vi "modbusRTU.vi"() -> ()   [LabVIEW 2019]
uses:
  <vilib>/Modbus/master/Create Master Instance (Serial).vi
  <vilib>/Modbus/master/Modbus Master.lvclass
panel:
  in  "Limpar":bool
  out "?":T1(graph)
  in  "Reset Button":bool
  out "modo (short)":enum16{"short", "long"}(ring) caption="Modo (16 ou 32b)"
  out "sistema 01":enum16{"sistema 01"}(ring) caption="Tipo do sistema"
  out "freq nom":enum16{"50 hz", "60 hz"}(ring) caption="Freq nominal"
  out "formato dado":T2(ring) caption="Formato dado"
  out "polaridade tc":enum16{"(+)", "(-)"}(ring) caption="Polaridade sensor"
  out "Gauge 2 Baud rate":u16(knob) caption="Baud rate" scale=1.0..8.0
  out "Freq instântanea":sgl
  out "Energia ativa total":sgl caption="Energia total kWh" format="%#.4f"
  out "Pot aparente fase A":sgl
  out "Pot reativa fase A":sgl
  out "Pot ativa fase A":sgl
  out "FP fase A":sgl
  out "Corrente fase A":sgl
  out "Tensão fase A":sgl
  out "estado saida IO2":bool caption="Estado saída I/O2"
  in  "holding register value input":u16 caption="Valor\nholding register"
  in  "holding register address":u16(ring) caption="Endereço\nholding register" items=["SPLL"=26, "SPHL"=27, "Type"=43, "Ctrl"=46, "Act"=48, "Atun"=49, "Unit"=67]
  out "SPHL":dbl
  out "SPLL":dbl
  in  "Write Button":bool
  out "Horizontal Pointer Slide Pb":dbl caption="Pb"
  out "Horizontal Pointer Slide Ir":dbl caption="Ir"
  out "Horizontal Pointer Slide 1 Dt":dbl caption="Dt"
  in  "Boolean Run":bool caption="Run"
  out "Gauge Baud rate":u16(knob) caption="Baud rate" scale=0.0..6.0
  in  "exit button":bool
  out "unit ID (nó)":u16 caption="Unit ID (nó)"
  out "Thermometer PV":dbl(slide) caption="PV - Temperatura" scale=0.0..300.0
  out "Unit":enum16{"ºC", "ºF"}(ring)
  out "Atun":T3(ring)
  out "Act":enum16{"rE", "d Ir", ""}(ring)
  out "Run":u16
  out "Ctrl":enum16{"Man", "Auto"}(ring)
  out "Addr (nó)":u16
  out "Type sensor":enum16{"", "tc K"}(ring) caption="Type"
  out "MV":u16(slide) caption="MV \n   ação \n     de \ncontrole" scale=0.0..100.0
  in  "stop button":bool
  in  "start button":bool
  in  "modo Modbus":enum16{"RTU", "ASCII"}(ring)
  in  "VISA resource name \nCOM port":refnum<visa-resource-name>="COM4"
  in  "parity bit":u16(ring)=2 caption="bit de paridade" items=["None", "Odd", "Even"]
  in  "flow control":u16(ring) items=["None", "XON/XOFF", "RTS/CTS", "XON/XOFF & RTS/CTS", "DTR/DSR", "XON/XOFF & DTR/DSR"]
  in  "baud rate":u32(ring)=9600 items=["1200"=1200, "2400"=2400, "4800"=4800, "9600"=9600, "19200"=19200, "57600"=57600]
  in  "holding register value SP":u16 caption="Setpoint (SP)"
  # "COMUNICAÇÃO ON/OFF"
  # "CONTROLADOR PID N1200"
  # "MULTIMEDIDOR M-200"
  # "VALORES REFERÊNCIA"
  # "Reading holding \n    registers (03)"
  # "Reading input \n  registers (04)"
  # "167 ºC"
  # "220 Vca"
  # "0,13 A"
  # "FP 0,99"
  # "Writing single \n  registers (06)"
  # "*Valores de referência do sistema sem controle de temperatura"
  # "Reading coils (01)"
  # "MESTRE \nMODBUS  RTU"
  # "Reading holding registers (03)"
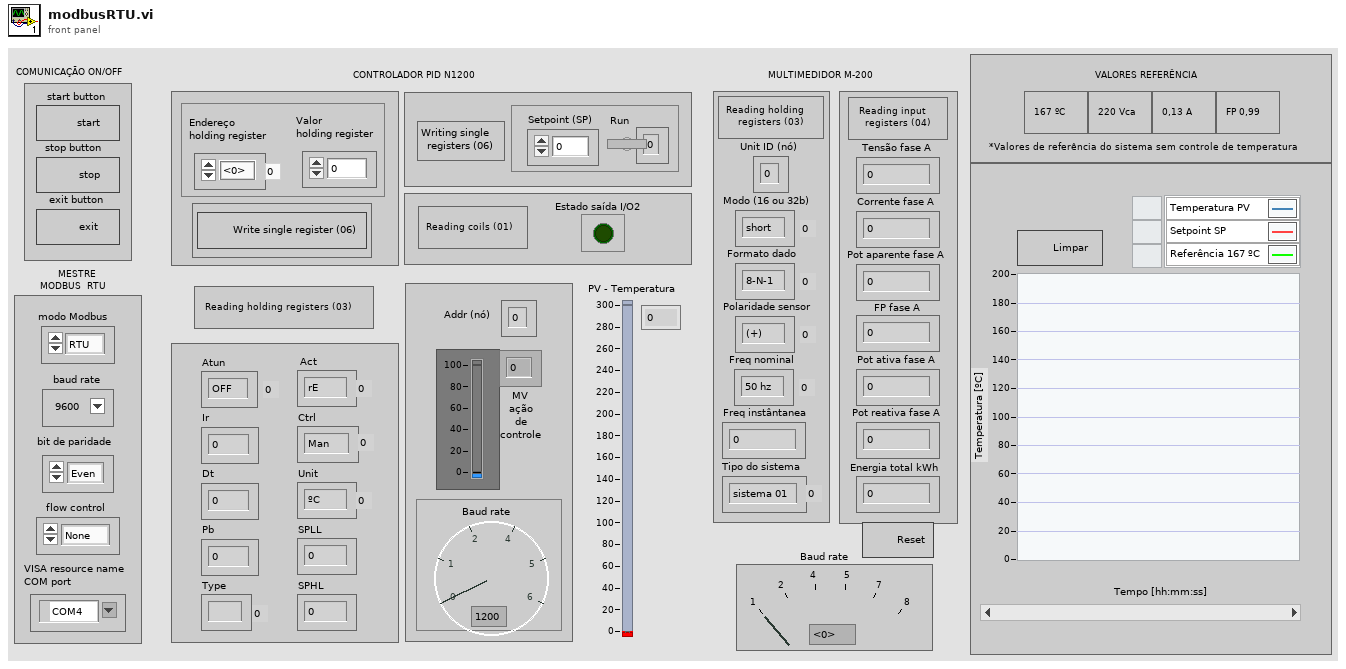
[diagram p1: front panel]
types:
  T1 = cluster{dbl, "y":u16, "holding register value SP":u16}
  T2 = enum16{"8-N-1", "8-N-2", "8-E-1", "8-E-2", "8-O-1", "8-O-2"}
  T3 = enum16{"OFF", "FAST", "FULL", "SELF", "RSELF", "TGHT"}
  T4 = cluster{dbl, "y":u16, "holding register value SP":u16}[]
  T5 = cluster{dbl, "holding register value SP":u16, "y":u16}
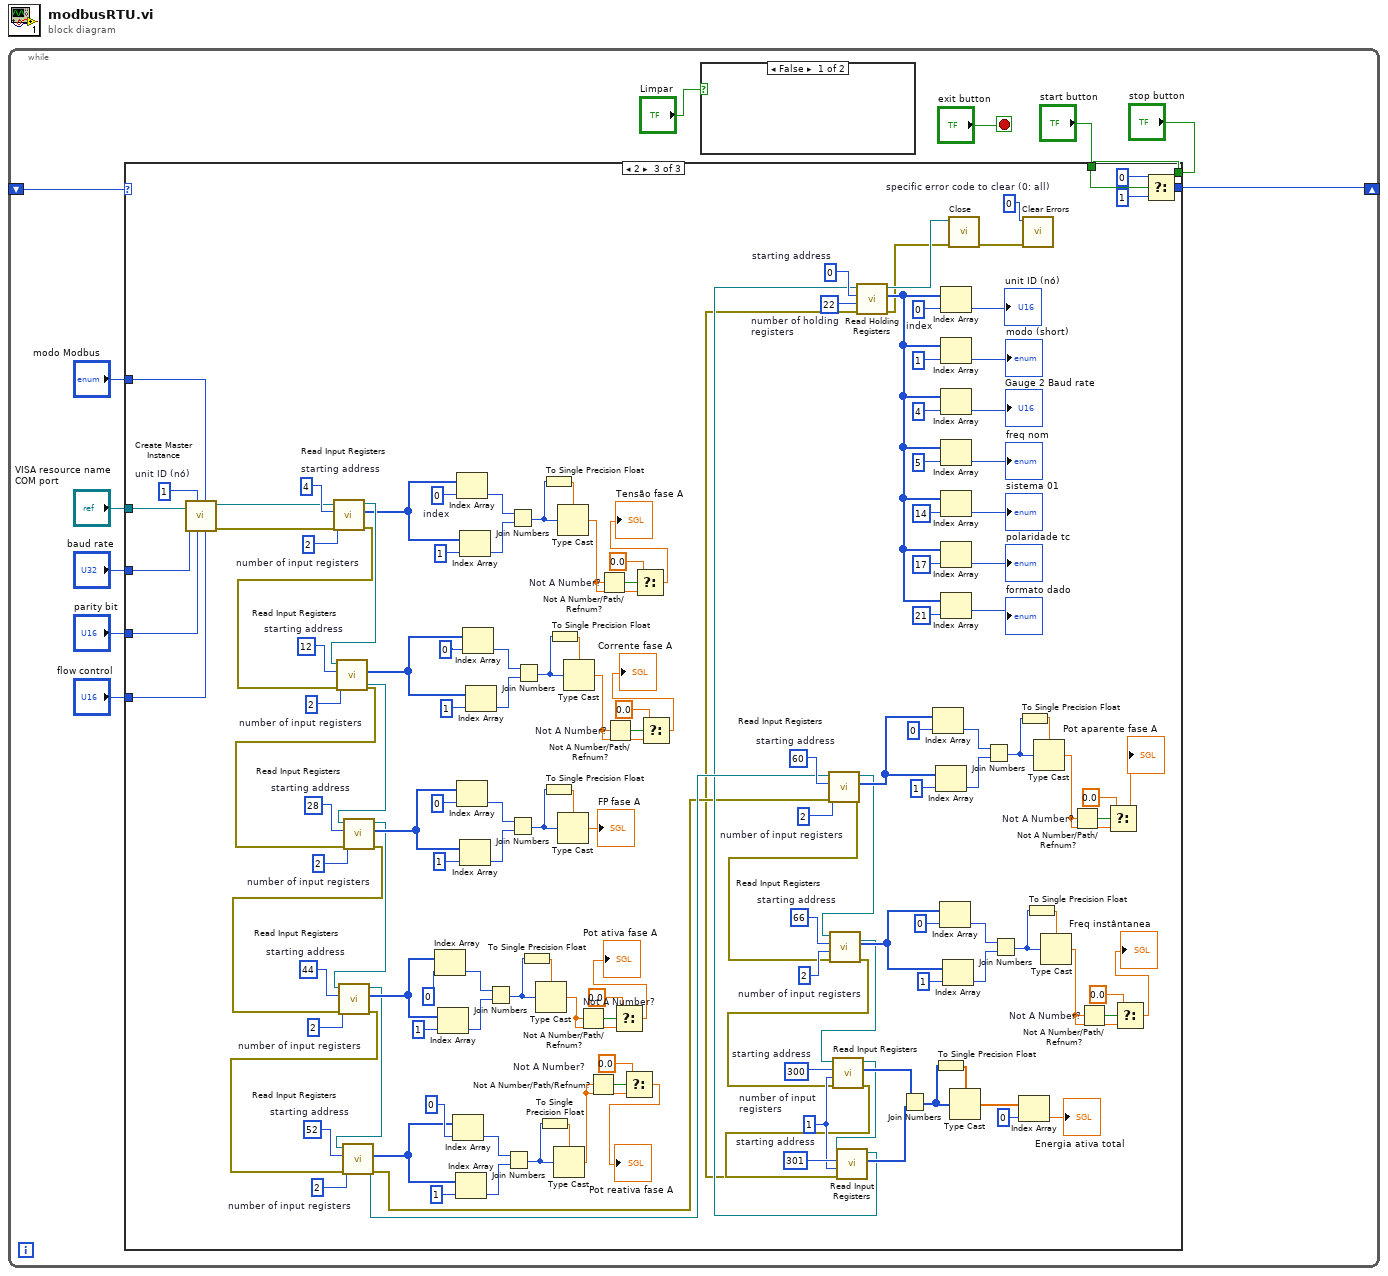
[diagram p0: block diagram]
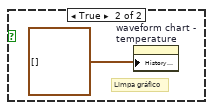
[diagram p2: hidden frame]
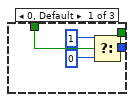
[diagram p3: hidden frame]
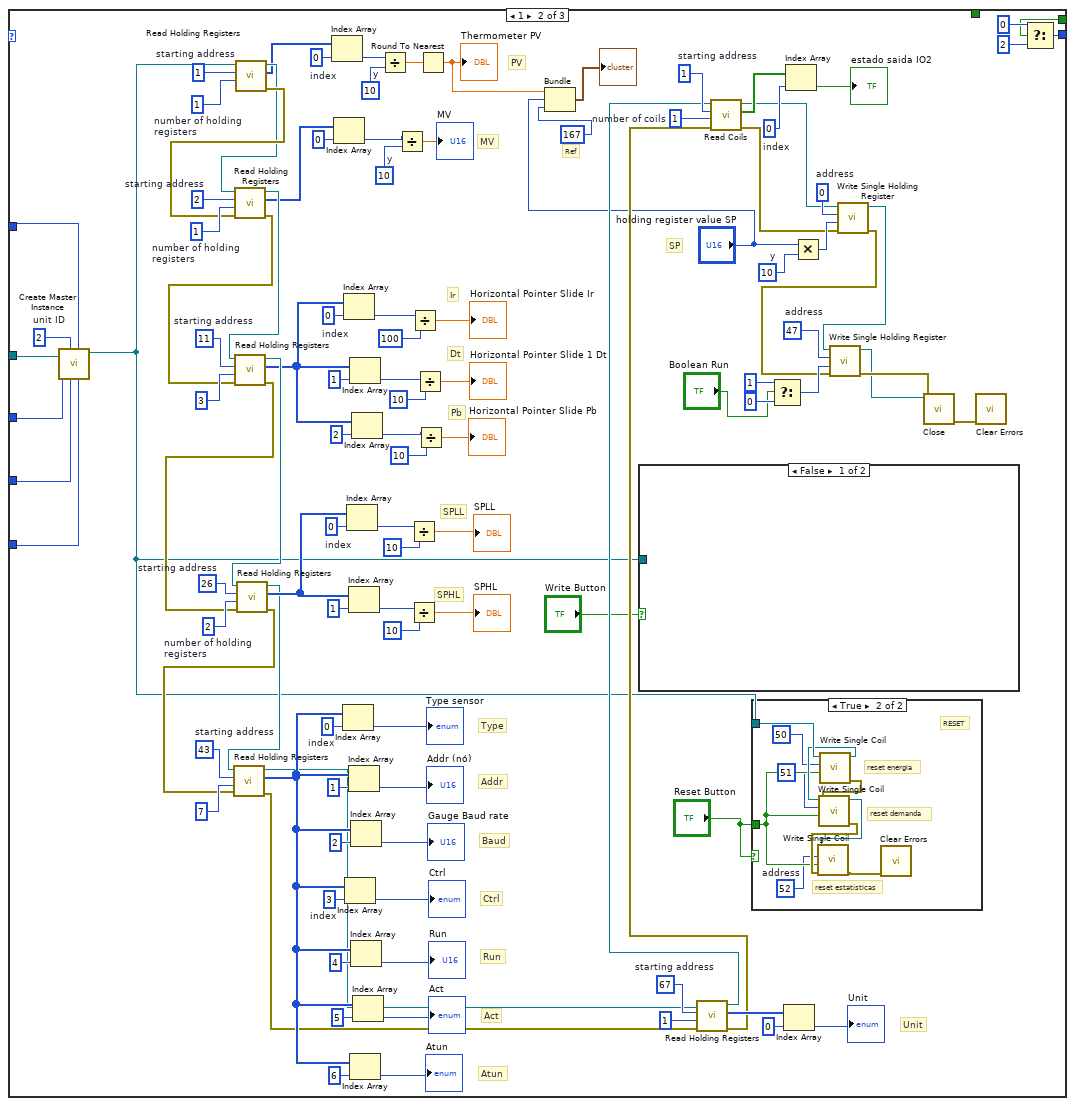
[diagram p4: hidden frame]
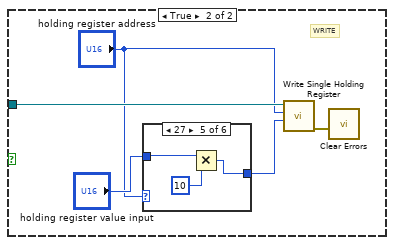
[diagram p6: hidden frame]
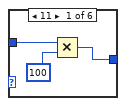
[diagram p7: hidden frame]
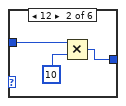
[diagram p8: hidden frame]
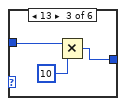
[diagram p9: hidden frame]
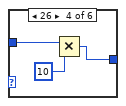
[diagram p10: hidden frame]
diagram:
  n1 = while {
    shift-right: [w10] -> _
    shift-left: _ -> [w11]
    stop <- "exit button" stop-if-true
    n2 = case shown="2" w11 {
      tunnel: [w16 w120 w303] -> w10
      tunnel: "stop button" -> [_ w119 w302]
      tunnel: "modo Modbus" -> [_ w118 w301]
      tunnel: "VISA resource name \nCOM port" -> [_ w117 w300]
      tunnel: "parity bit" -> [_ w115 w299]
      tunnel: "flow control" -> [_ w114 w298]
      tunnel: "baud rate" -> [_ w116 w297]
      tunnel: "start button" -> [w13 _ _]
      frame 0, Default {
        n3 = Select(t=1, s=w13, f=0) -> (s? t:f=w16:i32)
      }
      frame 1 {
        w29 = u16 1  # number of holding registers
        w30 = u16 1  # starting address
        w49 = 0  # index
        w52 = u16 1  # number of coils
        w53 = u16 1  # starting address
        w62 = u16 47  # address
        w66 = u16 10  # y
        w77 = u8 2  # unit ID
        w81 = u16 67  # starting address
        w91 = 3  # index
        w96 = 0  # index
        w98 = u16 43  # starting address
        w102 = 0  # index
        w99 = u16 2  # number of holding registers
        w103 = u16 26  # starting address
        w106 = 0  # index
        w108 = u16 11  # starting address
        w111 = 0  # index
        w112 = u16 10  # y
        w113 = u16 10  # y
        w125 = u16 1  # number of holding registers
        w126 = u16 2  # starting address
        w127 = u16 0  # address
        # "Ref"
        # "Unit"
        # "Atun"
        # "Act"
        # "Run"
        # "Ctrl"
        # "Baud"
        # "Addr"
        # "Type"
        # "SPHL"
        # "SPLL"
        # "Pb"
        # "Dt"
        # "Ir"
        # "MV"
        # "PV"
        # "SP"
        n4 = call-poly <vilib>:"Create Master Instance.vi"("flow control (None)"=w114, "serial type"=w118, "parity (Even)"=w115, "unit ID"=w77, "baud rate (9600)"=w116, "VISA resource name"=w117) -> ("serial master instance"=w22:refnum<class "Modbus Master.lvclass">)  [unwired: 4 in, 1 out]
        n5 = call-dynamic "Read Holding Registers.vi"("number of holding registers"=w29, "starting address"=w30, "Modbus master in"=w22) -> ("error out"=w28:errorcluster, "register values"=w23:u16[], "Modbus master out"=w27:refnum<class "Modbus Master.lvclass">)  [unwired: 6 in]
        n6 = call-dynamic "Read Holding Registers.vi"("error in (no error)"=w28, "number of holding registers"=w125, "starting address"=w126, "Modbus master in"=w27) -> ("error out"=w40:errorcluster, "register values"=w24:u16[], "Modbus master out"=w26:refnum<class "Modbus Master.lvclass">)  [unwired: 5 in]
        n7 = call-dynamic "Read Holding Registers.vi"("error in (no error)"=w40, "number of holding registers"=u16 3, "starting address"=w108, "Modbus master in"=w26) -> ("error out"=w39:errorcluster, "register values"=w25:u16[], "Modbus master out"=w46:refnum<class "Modbus Master.lvclass">)  [unwired: 5 in]
        n8 = call-dynamic "Read Holding Registers.vi"("error in (no error)"=w39, "number of holding registers"=w99, "starting address"=w103, "Modbus master in"=w46) -> ("error out"=w38:errorcluster, "register values"=w100:u16[], "Modbus master out"=w45:refnum<class "Modbus Master.lvclass">)  [unwired: 5 in]
        n9 = call-dynamic "Read Holding Registers.vi"("error in (no error)"=w38, "number of holding registers"=u16 7, "starting address"=w98, "Modbus master in"=w45) -> ("error out"=w37:errorcluster, "register values"=w83:u16[], "Modbus master out"=w44:refnum<class "Modbus Master.lvclass">)  [unwired: 5 in]
        n10 = Index Array "Index Array"(array=w23, index=w111) -> (element=w110:u16)
        n11 = Index Array(array=w24, index=0) -> (element=w65:u16)
        n12 = Index Array "Index Array"(array=w83, index=w96) -> (element=→"Type sensor":u16)
        n13 = Index Array "Index Array"(array=w25, index=w106) -> (element=w76:u16)
        n14 = Index Array(array=w83, index=w91) -> (element=→"Ctrl":u16)
        n15 = Index Array "Index Array"(array=w100, index=w102) -> (element=w69:u16)
        n16 = Index Array(array=w100, index=1) -> (element=w67:u16)
        n17 = Index Array(array=w83, index=1) -> (element=→"Addr (nó)":u16)
        n18 = Index Array(array=w25, index=1) -> (element=w73:u16)
        n19 = Index Array(array=w83, index=6) -> (element=→"Atun":u16)
        n20 = Index Array(array=w83, index=2) -> (element=→"Gauge Baud rate":u16)
        n21 = Index Array(array=w83, index=4) -> (element=→"Run":u16)
        n22 = Index Array(array=w25, index=2) -> (element=w71:u16)
        n23 = Index Array(array=w83, index=5) -> (element=→"Act":u16)
        n24 = Divide(x=w110, y=w112) -> (x/y=w123:dbl)
        n25 = Divide(x=w65, y=w66) -> (x/y=→"MV":dbl)
        n26 = Divide(x=w69, y=u16 10) -> (x/y=→"SPLL":dbl)
        n27 = Divide(x=w67, y=u16 10) -> (x/y=→"SPHL":dbl)
        n28 = Divide(x=w76, y=u16 100) -> (x/y=→"Horizontal Pointer Slide Ir":dbl)
        n29 = Divide(x=w73, y=u16 10) -> (x/y=→"Horizontal Pointer Slide 1 Dt":dbl)
        n30 = Divide(x=w71, y=u16 10) -> (x/y=→"Horizontal Pointer Slide Pb":dbl)
        n31 = Round To Nearest(number=w123) -> (nearest integer value=w20:dbl)
        "Thermometer PV" <- w20
        n32 = Bundle(w20, "holding register value SP"="holding register value SP", "y"=u16 167) -> (→"?":T5)  [unwired: 1 in]
        n33 = case shown="False" "Write Button" {
          tunnel: w22 -> [_ w141]
          frame False {
          }
          frame True {
            # "WRITE"
            n34 = case shown="27" "holding register address" {
              tunnel: [w144 w146 w149 w152 w155 w158] -> w140
              tunnel: "holding register value input" -> [w143 w147 w150 w153 w156 w158]
              frame 11 {
                n35 = Multiply(x=w143, y=u16 100) -> (x*y=w144:u16)
              }
              frame 12 {
                n36 = Multiply(x=w147, y=u16 10) -> (x*y=w146:u16)
              }
              frame 13 {
                n37 = Multiply(x=w150, y=u16 10) -> (x*y=w149:u16)
              }
              frame 26 {
                n38 = Multiply(x=w153, y=u16 10) -> (x*y=w152:u16)
              }
              frame 27 {
                n39 = Multiply(x=w156, y=u16 10) -> (x*y=w155:u16)
              }
              frame Default {
              }
            }
            n40 = call-dynamic "Write Single Holding Register.vi"("holding register value"=w140, "address"="holding register address", "Modbus master in"=w141) -> ("error out"=w142:errorcluster)  [unwired: 7 in, 1 out]
            n41 = call <vilib>:"Clear Errors.vi"("error in (no error)"=w142) -> ()  [unwired: 5 in, 2 out]
          }
        }
        n42 = call-dynamic "Read Holding Registers.vi"("error in (no error)"=w37, "number of holding registers"=u16 1, "starting address"=w81, "Modbus master in"=w44) -> ("error out"=w35:errorcluster, "register values"=w79:u16[], "Modbus master out"=w36:refnum<class "Modbus Master.lvclass">)  [unwired: 5 in]
        n43 = call-dynamic "Read Coils.vi"("error in (no error)"=w35, "number of coils"=w52, "starting address"=w53, "Modbus master in"=w36) -> ("error out"=w41:errorcluster, "coil values"=w50:bool[], "Modbus master out"=w47:refnum<class "Modbus Master.lvclass">)  [unwired: 5 in]
        n44 = case shown="True" "Reset Button" {
          tunnel: w22 -> [_ w134]
          tunnel: "Reset Button" -> [_ w131]
          frame False {
          }
          frame True {
            w130 = u16 52  # address
            # "RESET"
            # "reset estatísticas"
            # "reset demanda"
            # "reset energia"
            n45 = call-dynamic "Write Single Coil.vi"("coil value"=w131, "address"=u16 50, "Modbus master in"=w134) -> ("error out"=w137:errorcluster, "Modbus master out"=w133:refnum<class "Modbus Master.lvclass">)  [unwired: 7 in]
            n46 = call-dynamic "Write Single Coil.vi"("error in (no error)"=w137, "coil value"=w131, "address"=u16 51, "Modbus master in"=w133) -> ("error out"=w136:errorcluster, "Modbus master out"=w132:refnum<class "Modbus Master.lvclass">)  [unwired: 6 in]
            n47 = call-dynamic "Write Single Coil.vi"("error in (no error)"=w136, "coil value"=w131, "address"=w130, "Modbus master in"=w132) -> ("error out"=w135:errorcluster)  [unwired: 6 in, 1 out]
            n48 = call <vilib>:"Clear Errors.vi"("error in (no error)"=w135) -> ()  [unwired: 5 in, 2 out]
          }
        }
        n49 = Select(t=u16 1, s="Boolean Run", f=u16 0) -> (s? t:f=w59:u16)
        n50 = Index Array(array=w79, index=0) -> (element=→"Unit":u16)
        n51 = Index Array "Index Array"(array=w50, index=w49) -> (element=→"estado saida IO2":bool)
        n52 = Multiply(x="holding register value SP", y=w113) -> (x*y=w124:u16)
        n53 = call-dynamic "Write Single Holding Register.vi"("error in (no error)"=w41, "holding register value"=w124, "address"=w127, "Modbus master in"=w47) -> ("error out"=w42:errorcluster, "Modbus master out"=w51:refnum<class "Modbus Master.lvclass">)  [unwired: 6 in]
        n54 = call-dynamic "Write Single Holding Register.vi"("error in (no error)"=w42, "holding register value"=w59, "address"=w62, "Modbus master in"=w51) -> ("error out"=w34:errorcluster, "Modbus master out"=w33:refnum<class "Modbus Master.lvclass">)  [unwired: 6 in]
        n55 = call-dynamic "Close.vi"("error in (no error)"=w34, "Modbus master in"=w33) -> ("error out"=w43:errorcluster)  [unwired: 9 in]
        n56 = call <vilib>:"Clear Errors.vi"("error in (no error)"=w43) -> ()  [unwired: 5 in, 2 out]
        n57 = Select(t=0, s=w119, f=2) -> (s? t:f=w120:i32)
      }
      frame 2 {
        w189 = 0  # specific error code to clear (0: all)
        w222 = u16 2  # number of input registers
        w223 = u16 66  # starting address
        w228 = u16 2  # number of input registers
        w229 = u16 60  # starting address
        w230 = u16 2  # number of input registers
        w231 = u16 52  # starting address
        w232 = u16 2  # number of input registers
        w233 = u16 44  # starting address
        w234 = u16 2  # number of input registers
        w235 = u16 28  # starting address
        w236 = u16 2  # number of input registers
        w237 = u16 12  # starting address
        w246 = u16 301  # starting address
        w247 = u16 300  # starting address
        w238 = u16 1  # number of input registers
        w282 = 0  # index
        w285 = u16 2  # number of input registers
        w286 = u16 4  # starting address
        w294 = u8 1  # unit ID (nó)
        w296 = 0  # index
        w307 = u16 0  # starting address
        w306 = u16 22  # number of holding registers
        n58 = call-poly <vilib>:"Create Master Instance.vi"("flow control (None)"=w298, "serial type"=w301, "parity (Even)"=w299, "unit ID"=w294, "baud rate (9600)"=w297, "VISA resource name"=w300) -> ("error out"=w201:errorcluster, "serial master instance"=w203:refnum<class "Modbus Master.lvclass">)  [unwired: 4 in]
        n59 = call-dynamic "Read Input Registers.vi"("error in (no error)"=w201, "number of input registers"=w285, "starting address"=w286, "Modbus master in"=w203) -> ("error out"=w200:errorcluster, "register values"=w225:u16[], "Modbus master out"=w227:refnum<class "Modbus Master.lvclass">)  [unwired: 5 in]
        n60 = call-dynamic "Read Input Registers.vi"("error in (no error)"=w200, "number of input registers"=w236, "starting address"=w237, "Modbus master in"=w227) -> ("error out"=w199:errorcluster, "register values"=w212:u16[], "Modbus master out"=w226:refnum<class "Modbus Master.lvclass">)  [unwired: 5 in]
        n61 = call-dynamic "Read Input Registers.vi"("error in (no error)"=w199, "number of input registers"=w234, "starting address"=w235, "Modbus master in"=w226) -> ("error out"=w198:errorcluster, "register values"=w213:u16[], "Modbus master out"=w210:refnum<class "Modbus Master.lvclass">)  [unwired: 5 in]
        n62 = call-dynamic "Read Input Registers.vi"("error in (no error)"=w198, "number of input registers"=w232, "starting address"=w233, "Modbus master in"=w210) -> ("error out"=w197:errorcluster, "register values"=w214:u16[], "Modbus master out"=w209:refnum<class "Modbus Master.lvclass">)  [unwired: 5 in]
        n63 = call-dynamic "Read Input Registers.vi"("error in (no error)"=w197, "number of input registers"=w230, "starting address"=w231, "Modbus master in"=w209) -> ("error out"=w196:errorcluster, "register values"=w211:u16[], "Modbus master out"=w208:refnum<class "Modbus Master.lvclass">)  [unwired: 5 in]
        n64 = Index Array(array=w214, index=0) -> (element=w262:u16)
        n65 = Index Array(array=w214, index=1) -> (element=w260:u16)
        n66 = Index Array(array=w211, index=0) -> (element=w256:u16)
        n67 = Index Array(array=w211, index=1) -> (element=w254:u16)
        n68 = Index Array "Index Array"(array=w225, index=w282) -> (element=w281:u16)
        n69 = Index Array(array=w213, index=0) -> (element=w269:u16)
        n70 = Index Array(array=w225, index=1) -> (element=w279:u16)
        n71 = Index Array(array=w213, index=1) -> (element=w267:u16)
        n72 = Index Array(array=w212, index=0) -> (element=w275:u16)
        n73 = Index Array(array=w212, index=1) -> (element=w273:u16)
        n74 = Join Numbers(hi=w262, lo=w260) -> ((hi.lo)=w264:u32)
        n75 = Join Numbers(hi=w256, lo=w254) -> ((hi.lo)=w258:u32)
        n76 = Join Numbers(hi=w281, lo=w279) -> ((hi.lo)=w283:u32)
        n77 = Join Numbers(hi=w269, lo=w267) -> ((hi.lo)=w271:u32)
        n78 = Join Numbers(hi=w275, lo=w273) -> ((hi.lo)=w277:u32)
        n79 = To Single Precision Float(number=w264) -> (single precision float=w265:sgl)
        n80 = Type Cast(type=w265, x=w264) -> (*(type *) &x=w172:sgl)
        n81 = To Single Precision Float(number=w258) -> (single precision float=w259:sgl)
        n82 = To Single Precision Float(number=w283) -> (single precision float=w284:sgl)
        n83 = To Single Precision Float(number=w271) -> (single precision float=w272:sgl)
        n84 = To Single Precision Float(number=w277) -> (single precision float=w278:sgl)
        n85 = Type Cast(type=w259, x=w258) -> (*(type *) &x=w167:sgl)
        n86 = Type Cast(type=w284, x=w283) -> (*(type *) &x=w180:sgl)
        n87 = Type Cast(type=w272, x=w271) -> (*(type *) &x=→"FP fase A":sgl)
        n88 = Type Cast(type=w278, x=w277) -> (*(type *) &x=w176:sgl)
        n89 = Not A Number/Path/Refnum? "Not A Number?"(number/path/refnum=w172) -> (NaN/Path/Refnum?=w174:bool)
        n90 = Not A Number/Path/Refnum? "Not A Number?"(number/path/refnum=w167) -> (NaN/Path/Refnum?=w170:bool)
        n91 = Not A Number/Path/Refnum? "Not A Number?"(number/path/refnum=w180) -> (NaN/Path/Refnum?=w182:bool)
        n92 = Not A Number/Path/Refnum? "Not A Number?"(number/path/refnum=w176) -> (NaN/Path/Refnum?=w178:bool)
        n93 = Select(t=0.0, s=w174, f=w172) -> (s? t:f=→"Pot ativa fase A":dbl)
        n94 = Select(t=0.0, s=w170, f=w167) -> (s? t:f=→"Pot reativa fase A":dbl)
        n95 = Select(t=0.0, s=w182, f=w180) -> (s? t:f=→"Tensão fase A":dbl)
        n96 = Select(t=0.0, s=w178, f=w176) -> (s? t:f=→"Corrente fase A":dbl)
        n97 = call-dynamic "Read Input Registers.vi"("error in (no error)"=w196, "number of input registers"=w228, "starting address"=w229, "Modbus master in"=w208) -> ("error out"=w195:errorcluster, "register values"=w224:u16[], "Modbus master out"=w207:refnum<class "Modbus Master.lvclass">)  [unwired: 5 in]
        n98 = call-dynamic "Read Input Registers.vi"("error in (no error)"=w195, "number of input registers"=w222, "starting address"=w223, "Modbus master in"=w207) -> ("error out"=w194:errorcluster, "register values"=w215:u16[], "Modbus master out"=w206:refnum<class "Modbus Master.lvclass">)  [unwired: 5 in]
        n99 = call-dynamic "Read Input Registers.vi"("error in (no error)"=w194, "number of input registers"=w238, "starting address"=w247, "Modbus master in"=w206) -> ("error out"=w193:errorcluster, "register values"=w245:u16[], "Modbus master out"=w205:refnum<class "Modbus Master.lvclass">)  [unwired: 5 in]
        n100 = call-dynamic "Read Input Registers.vi"("error in (no error)"=w193, "number of input registers"=w238, "starting address"=w246, "Modbus master in"=w205) -> ("error out"=w192:errorcluster, "register values"=w244:u16[], "Modbus master out"=w204:refnum<class "Modbus Master.lvclass">)  [unwired: 5 in]
        n101 = call-dynamic "Read Holding Registers.vi"("error in (no error)"=w192, "number of holding registers"=w306, "starting address"=w307, "Modbus master in"=w204) -> ("error out"=w191:errorcluster, "register values"=w287:u16[], "Modbus master out"=w202:refnum<class "Modbus Master.lvclass">)  [unwired: 5 in]
        n102 = Join Numbers(hi=w245, lo=w244) -> ((hi.lo)=w242:u32[])
        n103 = Index Array(array=w224, index=0) -> (element=w250:u16)
        n104 = Index Array(array=w224, index=1) -> (element=w248:u16)
        n105 = To Single Precision Float(number=w242) -> (single precision float=w243:sgl[])
        n106 = Index Array(array=w215, index=0) -> (element=w218:u16)
        n107 = Index Array "Index Array"(array=w287, index=w296) -> (element=→"unit ID (nó)":u16)
        n108 = Index Array(array=w287, index=1) -> (element=→"modo (short)":u16)
        n109 = Index Array(array=w287, index=4) -> (element=→"Gauge 2 Baud rate":u16)
        n110 = Index Array(array=w287, index=5) -> (element=→"freq nom":u16)
        n111 = Index Array(array=w287, index=14) -> (element=→"sistema 01":u16)
        n112 = Index Array(array=w287, index=17) -> (element=→"polaridade tc":u16)
        n113 = Index Array(array=w287, index=21) -> (element=→"formato dado":u16)
        n114 = Index Array(array=w215, index=1) -> (element=w216:u16)
        n115 = call-dynamic "Close.vi"("error in (no error)"=w191, "Modbus master in"=w202) -> ("error out"=w190:errorcluster)  [unwired: 9 in]
        n116 = Type Cast(type=w243, x=w242) -> (*(type *) &x=w241:sgl[])
        n117 = Join Numbers(hi=w250, lo=w248) -> ((hi.lo)=w252:u32)
        n118 = Join Numbers(hi=w218, lo=w216) -> ((hi.lo)=w220:u32)
        n119 = Index Array(array=w241, index=0) -> (element=→"Energia ativa total":sgl)
        n120 = To Single Precision Float(number=w252) -> (single precision float=w253:sgl)
        n121 = call <vilib>:"Clear Errors.vi"("error in (no error)"=w190, "specific error code to clear (0: all)"=w189) -> ()  [unwired: 4 in, 2 out]
        n122 = To Single Precision Float(number=w220) -> (single precision float=w221:sgl)
        n123 = Type Cast(type=w253, x=w252) -> (*(type *) &x=w159:sgl)
        n124 = Type Cast(type=w221, x=w220) -> (*(type *) &x=w163:sgl)
        n125 = Not A Number/Path/Refnum? "Not A Number?"(number/path/refnum=w159) -> (NaN/Path/Refnum?=w162:bool)
        n126 = Not A Number/Path/Refnum? "Not A Number?"(number/path/refnum=w163) -> (NaN/Path/Refnum?=w166:bool)
        n127 = Select(t=0.0, s=w162, f=w159) -> (s? t:f=→"Pot aparente fase A":dbl)
        n128 = Select(t=0.0, s=w166, f=w163) -> (s? t:f=→"Freq instântanea":dbl)
        n129 = Select(t=0, s=w302, f=1) -> (s? t:f=w303:i32)
      }
    }
    n130 = case shown="False" "Limpar" {
      frame False {
      }
      frame True {
        # "Limpa gráfico"
        n131 = property on="waveform chart - temperature" class="WFChart (strict)"("History Data"=T4 []) -> ()  [unwired: 2 in, 2 out]
      }
    }
  }
